vi "CameraSubVI.vi"() -> ()   [LabVIEW 2013]
uses:
  <vilib>/userdefined/High Color/IMAQdx.ctl
  <vilib>/vision/driver/NI_Vision_Acquisition_Software.lvlib
  <resource>/objmgr/imaqdx.rc
panel:
  in  "Video Modes":i32(listbox)=22
  out "Image":T1(plugin-control)
  in  "Camera Name":T2="cam0"
  in  "stop":bool
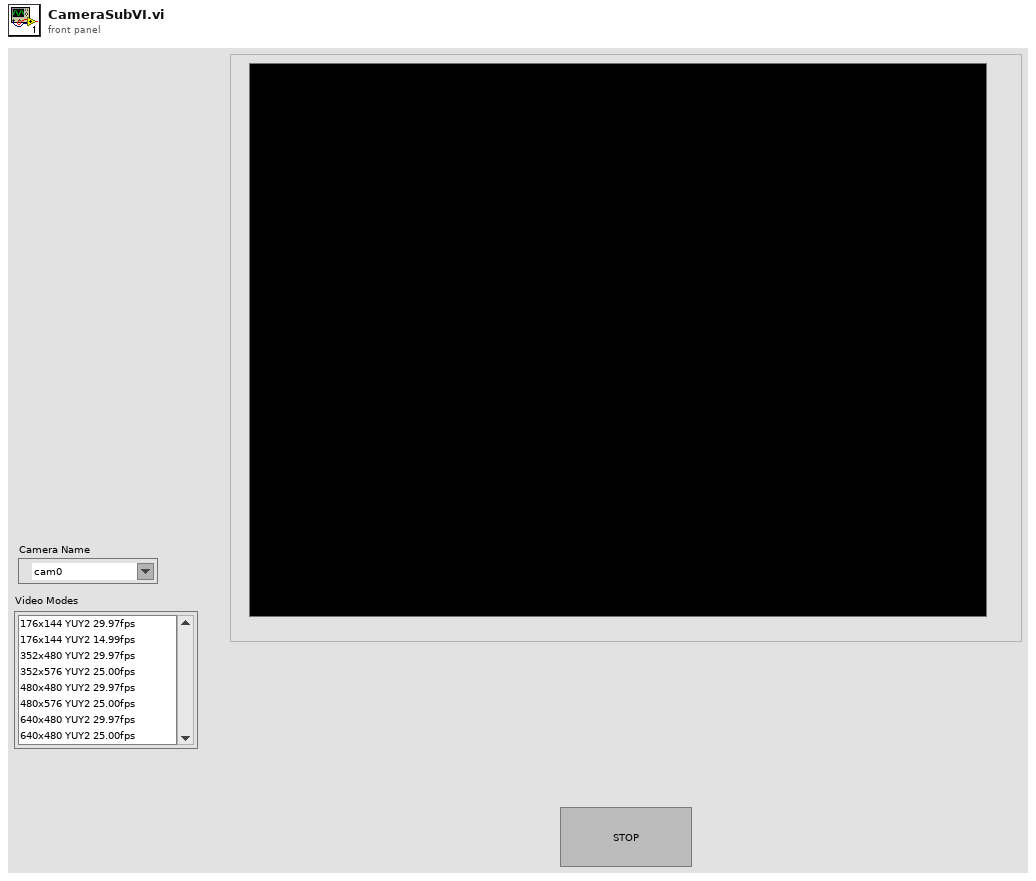
[diagram p1: front panel]
types:
  T1 = typedef "IMAQ Image.ctl" = refnum<image>
  T2 = typedef "IMAQdx.ctl" = refnum<k21>
  T3 = typedef "Image Type" = u32
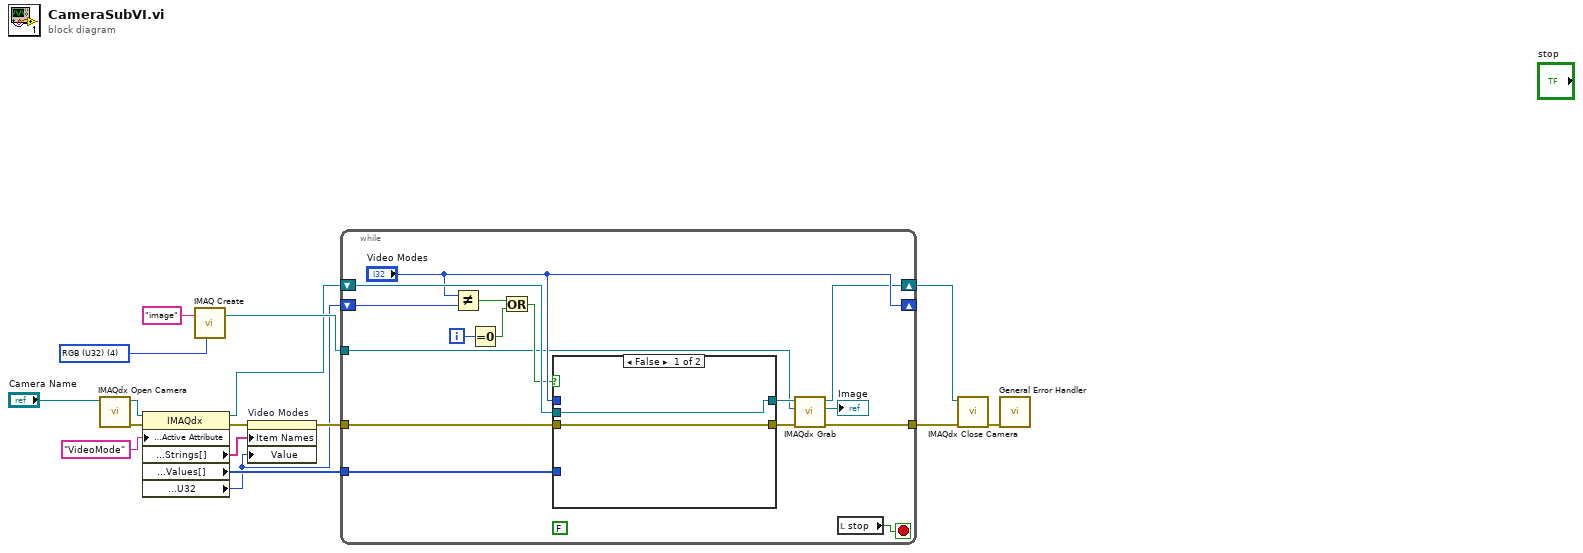
[diagram p0: block diagram]
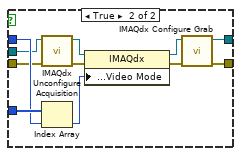
[diagram p2: hidden frame]
diagram:
  w1 = T3 4 items=["Grayscale (U8)", "Grayscale (I16)", "Grayscale (SGL)", "Complex (CSG)", "RGB (U32)", "HSL (U32)", "RGB (U64)", "Grayscale (U16)"] ("Image Type")
  n1 = call <vilib>:"IMAQdx Open Camera.vi"("Session In"="Camera Name") -> ("error out"=w7:errorcluster, "Session Out"=w10:T2)  [unwired: 2 in, 7 out]
  n2 = property class="IMAQdx"(reference=w10, error in=w7, "Camera Attributes:Active Attribute"="VideoMode" ("ActiveAttribute")) -> (reference out=w5:T2, error out=w6:errorcluster, "Camera Attributes:Enum:Strings[]"=w3:string[], "Camera Attributes:Enum:Values[]"=w8:u32[], "Camera Attributes:Value:U32"=w2:u32)
  n3 = call "IMAQ Create"("Image Name"="image", "Image Type"=w1) -> ("New Image"=w13:T1)  [unwired: 2 in, 2 out]
  n4 = property on="Video Modes" class="LstBox (strict)"(error in=w6, "Item Names"=w3, "Value"=w2) -> (error out=w4:errorcluster)  [unwired: 1 in, 1 out]
  n5 = while {
    tunnel: w8 -> [w30]
    shift-left: w2 -> [w29]
    shift-right: ["Video Modes"] -> _
    tunnel: w13 -> [w19]
    tunnel: w4 -> [w31]
    tunnel: [w21] -> w15
    shift-right: [w22] -> w12
    shift-left: w5 -> [w32]
    i -> [w18]
    stop <- w17 stop-if-true
    (unwired) FALSE
    n6 = Not Equal?(x="Video Modes", y=w29) -> (x != y?=w26:bool)
    n7 = Equal To 0?(x=w18) -> (x = 0?=w25:bool)
    n8 = Or(x=w26, y=w25) -> (x .or. y?=w27:bool)
    n9 = case shown="False" w27 {
      tunnel: w32 -> [w34 w43]
      tunnel: w31 -> [w33 w42]
      tunnel: [w34 w39] -> w23
      tunnel: [w33 w40] -> w24
      tunnel: w30 -> [_ w45]
      tunnel: "Video Modes" -> [_ w44]
      frame False {
      }
      frame True {
        n10 = call <vilib>:"IMAQdx Unconfigure Acquisition.vi"("error in"=w42, "Session In"=w43) -> ("error out"=w36:errorcluster, "Session Out"=w41:T2)  [unwired: 8 out]
        n11 = Index Array(array=w45, index=w44) -> (element=w35:u32)
        n12 = property class="IMAQdx"(reference=w41, error in=w36, "Acquisition Attributes:Video Mode"=w35) -> (reference out=w38:T2, error out=w37:errorcluster)
        n13 = call <vilib>:"IMAQdx Configure Grab.vi"("error in"=w37, "Session In"=w38) -> ("error out"=w40:errorcluster, "Session Out"=w39:T2)  [unwired: 1 in, 7 out]
      }
    }
    n14 = call <vilib>:"IMAQdx Grab.vi"("error in"=w24, "Image In"=w19, "Session In"=w23) -> ("error out"=w21:errorcluster, "Image Out"=→"Image":T1, "Session Out"=w22:T2)  [unwired: 1 in, 5 out]
    n15 = local read "stop"() -> (w17:bool)
  }
  n16 = call <vilib>:"IMAQdx Close Camera.vi"("error in"=w15, "Session In"=w12) -> ("error out"=w16:errorcluster)  [unwired: 9 out]
  n17 = call <vilib>:"General Error Handler.vi"("error in (no error)"=w16) -> ()  [unwired: 1 in, 14 out]
